vi "Take Measurement.vi"(8 "error in (no error)":errorcluster, 11 "SweepControl in":refnum<class "Sweep Control.lvclass">) -> (0 "error out":errorcluster, 3 "SweepControl":refnum<class "Sweep Control.lvclass">)   [LabVIEW 2019, in "Sweep Control.lvclass"]
uses:
  Sweep Control.lvclass
  <userlib>/LevyLab/Transport/Transport Server/Inst.Transport/Inst.Transport.lvclass
  <userlib>/LevyLab/Transport/Transport/Transport.lvclass
  <userlib>/LevyLab/Transport/Control Experiment/Control Experiment.lvclass
  <userlib>/LevyLab/Transport/Transport Server/Inst.Transport/Typedefs/Inst.Transport.Methods--Enum.ctl
  <userlib>/LevyLab/Transport/Transport Server/Inst.Transport/Typedefs/Inst.Transport.Status--Enum.ctl
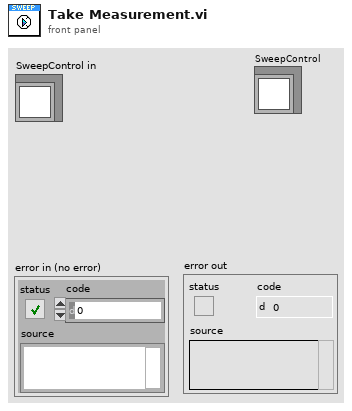
[diagram p1: front panel]
types:
  T1 = typedef "Sweep Control.lvclass/Enum - Experiments.ctl" = enum16{"LockinTime", "LockinSweep", "LockinDelayLine"}
  T2 = typedef "Inst.Transport.lvclass/Inst.Transport.Methods--Enum.ctl" = enum16{"LockinSweep", "LockinTime", "LockinTimeDelay"}
  T3 = typedef "Inst.Transport.lvclass/Inst.Transport.Status--Enum.ctl" = enum16{"idle", "running"}
  T4 = typedef "Transport.lvclass/Lockin_Sweep JSON--Cluster.ctl" = cluster{"initialWaitTime":dbl, "sweepTime":dbl, "Return to Start":bool, "sweepChannels":cluster{"Enable?":bool, "Channel":u16, "Start":dbl, "End":dbl, "Pattern":enum16{"Ramp /", "Ramp /\\", "Smooth Ramp _/", "Smooth Ramp _/\\_", "Table"}, "Table":dbl[]}[], "sweepTables":cluster{"Ch":i32, "Table":dbl[]}[]}
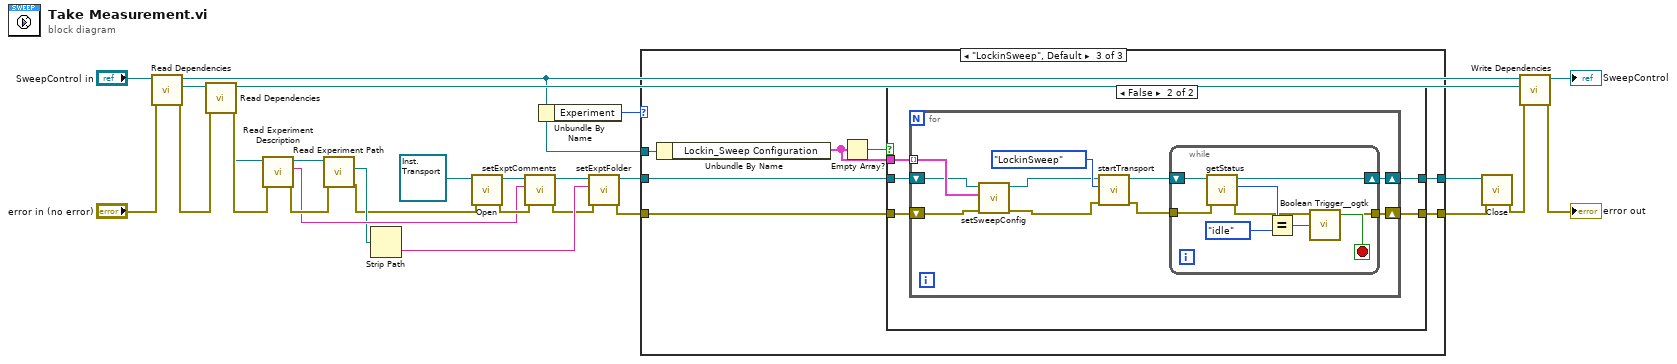
[diagram p0: block diagram]
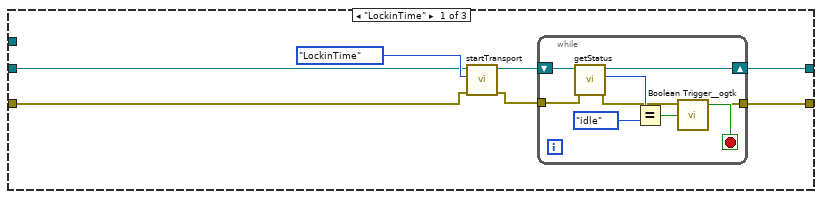
[diagram p2: hidden frame]
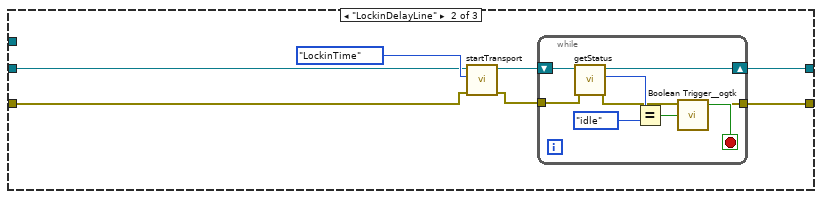
[diagram p3: hidden frame]
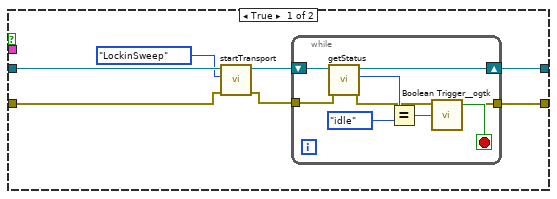
[diagram p4: hidden frame]
diagram:
  n1 = call <userlib>:"Read Dependencies.vi"("error in (no error)"="error in (no error)", "SweepControl in"="SweepControl in") -> ("error out"=w24:errorcluster, "Transport"=w23:refnum<class "Transport.lvclass">, "SweepControl out"=w1:refnum<class "Sweep Control.lvclass">)  [unwired: 7 in]
  n2 = call <userlib>:"Read Dependencies.vi"("error in (no error)"=w24, "Transport"=w23) -> ("error out"=w18:errorcluster, "C.E."=w17:refnum<class "Control Experiment.lvclass">, "Transport"=w22:refnum<class "Transport.lvclass">)  [unwired: 7 in]
  n3 = call <userlib>:"Read Experiment Description.vi"("error in (no error)"=w18, "Control Experiment in"=w17) -> ("error out"=w15:errorcluster, "Experiment Description"=w12:string, "Control Experiment out"=w16:refnum<class "Control Experiment.lvclass">)  [unwired: 7 in]
  n4 = call <userlib>:"Read Experiment Path.vi"("error in (no error)"=w15, "Control Experiment in"=w16) -> ("error out"=w7:errorcluster, "Experiment Path"=w11:path)  [unwired: 7 in, 1 out]
  n5 = Strip Path(path=w11) -> (name=w10:string)  [unwired: 1 out]
  n6 = call-dynamic "Open.vi"("error in (no error)"=w7, "Inst.Transport in"=refnum<class "Inst.Transport.lvclass"> refnum) -> ("error out"=w13:errorcluster, "Inst.Transport out"=w14:refnum<class "Inst.Transport.lvclass">)  [unwired: 8 in]
  n7 = call <userlib>:"setExptComments.vi"("error in (no error)"=w13, "comments"=w12, "Inst.Transport in"=w14) -> ("error out"=w8:errorcluster, "Inst.Transport out"=w9:refnum<class "Inst.Transport.lvclass">)  [unwired: 7 in]
  n8 = Unbundle By Name(w1) -> ("Experiment"=w27:T1)
  n9 = call <userlib>:"setExptFolder.vi"("error in (no error)"=w8, "folder"=w10, "Inst.Transport in"=w9) -> ("error out"=w2:errorcluster, "Inst.Transport out"=w3:refnum<class "Inst.Transport.lvclass">)  [unwired: 7 in]
  n10 = case shown="\"LockinSweep\", Default" w27 {
    tunnel: [w34 w49 w64] -> w6
    tunnel: [w33 w48 w63] -> w4
    tunnel: w3 -> [w29 w44 w62]
    tunnel: w2 -> [w28 w43 w61]
    tunnel: w1 -> [_ _ w60]
    frame "LockinTime" {
      n11 = call <userlib>:"startTransport.vi"("error in (no error)"=w28, "method"=Inst.Transport.Methods--Enum."LockinTime", "Inst.Transport in"=w29) -> ("error out"=w31:errorcluster, "Inst.Transport out"=w30:refnum<class "Inst.Transport.lvclass">)  [unwired: 7 in]
      n12 = while {
        tunnel: w31 -> [w42]
        shift-right: [w37] -> w34
        shift-left: w30 -> [w41]
        tunnel: [w35] -> w33
        stop <- w36 stop-if-true
        n13 = call <userlib>:"getStatus.vi"("error in (no error)"=w42, "Inst.Transport in"=w41) -> ("error out"=w35:errorcluster, "Status"=w40:T3, "Inst.Transport out"=w37:refnum<class "Inst.Transport.lvclass">)  [unwired: 7 in]
        n14 = Equal?(x=w40, y=Inst.Transport.Status--Enum."idle" ("Status")) -> (x = y?=w38:bool)
        n15 = call <userlib>:"Boolean Trigger__ogtk.vi"("Boolean Input"=w38) -> ("Rising Edge"=w36:bool)  [unwired: 1 in, 1 out]
      }
    }
    frame "LockinDelayLine" {
      n16 = call <userlib>:"startTransport.vi"("error in (no error)"=w43, "method"=Inst.Transport.Methods--Enum."LockinTime", "Inst.Transport in"=w44) -> ("error out"=w46:errorcluster, "Inst.Transport out"=w45:refnum<class "Inst.Transport.lvclass">)  [unwired: 7 in]
      n17 = while {
        tunnel: w46 -> [w57]
        shift-right: [w52] -> w49
        shift-left: w45 -> [w56]
        tunnel: [w50] -> w48
        stop <- w51 stop-if-true
        n18 = call <userlib>:"getStatus.vi"("error in (no error)"=w57, "Inst.Transport in"=w56) -> ("error out"=w50:errorcluster, "Status"=w55:T3, "Inst.Transport out"=w52:refnum<class "Inst.Transport.lvclass">)  [unwired: 7 in]
        n19 = Equal?(x=w55, y=Inst.Transport.Status--Enum."idle" ("Status")) -> (x = y?=w53:bool)
        n20 = call <userlib>:"Boolean Trigger__ogtk.vi"("Boolean Input"=w53) -> ("Rising Edge"=w51:bool)  [unwired: 1 in, 1 out]
      }
    }
    frame "LockinSweep", Default {
      n21 = Unbundle By Name(w60) -> ("Lockin_Sweep Configuration"=w58:T4[])
      n22 = Empty Array?(array=w58) -> (empty?=w59:bool)
      n23 = case shown="False" w59 {
        tunnel: [w71 w84] -> w64
        tunnel: [w70 w83] -> w63
        tunnel: w62 -> [w69 w82]
        tunnel: w61 -> [w68 w81]
        tunnel: w58 -> [_ w80]
        frame True {
          n24 = call <userlib>:"startTransport.vi"("error in (no error)"=w68, "method"=Inst.Transport.Methods--Enum."LockinSweep", "Inst.Transport in"=w69) -> ("error out"=w66:errorcluster, "Inst.Transport out"=w65:refnum<class "Inst.Transport.lvclass">)  [unwired: 7 in]
          n25 = while {
            tunnel: w66 -> [w79]
            shift-right: [w74] -> w71
            shift-left: w65 -> [w78]
            tunnel: [w72] -> w70
            stop <- w73 stop-if-true
            n26 = call <userlib>:"getStatus.vi"("error in (no error)"=w79, "Inst.Transport in"=w78) -> ("error out"=w72:errorcluster, "Status"=w77:T3, "Inst.Transport out"=w74:refnum<class "Inst.Transport.lvclass">)  [unwired: 7 in]
            n27 = Equal?(x=w77, y=Inst.Transport.Status--Enum."idle" ("Status")) -> (x = y?=w75:bool)
            n28 = call <userlib>:"Boolean Trigger__ogtk.vi"("Boolean Input"=w75) -> ("Rising Edge"=w73:bool)  [unwired: 1 in, 1 out]
          }
        }
        frame False {
          n29 = for {
            shift-right: [w94] -> w84
            shift-left: w82 -> [w88]
            shift-right: [w93] -> w83
            shift-left: w81 -> [w86]
            tunnel: w80 -> [w89] mode=indexing
            n30 = call <userlib>:"setSweepConfig.vi"("error in (no error)"=w86, "SweepConfig"=w89, "Inst.Transport in"=w88) -> ("error out"=w85:errorcluster, "Inst.Transport out"=w87:refnum<class "Inst.Transport.lvclass">)  [unwired: 7 in]
            n31 = call <userlib>:"startTransport.vi"("error in (no error)"=w85, "method"=Inst.Transport.Methods--Enum."LockinSweep", "Inst.Transport in"=w87) -> ("error out"=w91:errorcluster, "Inst.Transport out"=w90:refnum<class "Inst.Transport.lvclass">)  [unwired: 7 in]
            n32 = while {
              tunnel: w91 -> [w102]
              shift-right: [w97] -> w94
              shift-left: w90 -> [w101]
              tunnel: [w95] -> w93
              stop <- w96 stop-if-true
              n33 = call <userlib>:"getStatus.vi"("error in (no error)"=w102, "Inst.Transport in"=w101) -> ("error out"=w95:errorcluster, "Status"=w100:T3, "Inst.Transport out"=w97:refnum<class "Inst.Transport.lvclass">)  [unwired: 7 in]
              n34 = Equal?(x=w100, y=Inst.Transport.Status--Enum."idle" ("Status")) -> (x = y?=w98:bool)
              n35 = call <userlib>:"Boolean Trigger__ogtk.vi"("Boolean Input"=w98) -> ("Rising Edge"=w96:bool)  [unwired: 1 in, 1 out]
            }
          }
        }
      }
    }
  }
  n36 = call-dynamic "Close.vi"("error in (no error)"=w4, "Inst.Transport in"=w6) -> ("error out"=w20:errorcluster)  [unwired: 8 in, 1 out]
  n37 = call "Write Dependencies.vi"("error in (no error)"=w20, "Transport"=w22, "SweepControl in"=w1) -> ("error out"=→"error out":errorcluster, "SweepControl out"=→"SweepControl":refnum<class "Sweep Control.lvclass">)  [unwired: 7 in]
